vi "Host - Watchdog Init (SubVI).vi"(8 "error in":errorcluster, 11 "Pilot":bool) -> (0 "error out":errorcluster)   [LabVIEW 2021]
doc: "This vi initlize the watch Dog method . which used for the teh piolet and co-piolet communcation"
panel:
  out "Data out":i32
  out "Data":i32
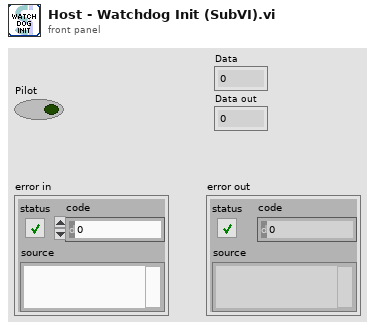
[diagram p1: front panel]
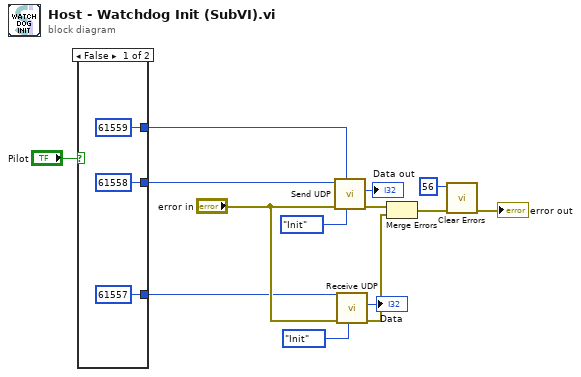
[diagram p0: block diagram]
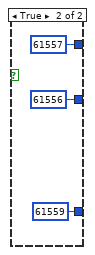
[diagram p2: hidden frame]
diagram:
  n1 = case shown="False" "Pilot" {
    tunnel: [u16 61559 ("remote port") u16 61557 ("remote port")] -> w5
    tunnel: [u16 61558 ("local port") u16 61556 ("local port")] -> w4
    tunnel: [u16 61557 ("receiver port") u16 61559 ("receiver port")] -> w3
    frame False {
    }
    frame True {
    }
  }
  n2 = call "Send UDP.vi"("Operation"=enum16{"Init", "Send", "Close"}."Init", "remote port"=w5, "error in"="error in", "local port"=w4) -> ("error out"=w9:errorcluster, "Data out"=→"Data out":i32)  [unwired: 6 in]
  n3 = call "Receive UDP.vi"("Operation"=enum16{"Init", "Receive", "Close"}."Init", "error in"="error in", "receiver port"=w3) -> ("error out"=w7:errorcluster, "Data"=→"Data":i32)  [unwired: 6 in, 1 out]
  n4 = Merge Errors(w9, w7) -> (w13:errorcluster)
  n5 = call <vilib>:"Clear Errors.vi"("error in (no error)"=w13, "specific error code to clear (0: all)"=56) -> ("error out"=→"error out":errorcluster)  [unwired: 4 in, 1 out]
